vi "Intake Loop.vi"   [LabVIEW 2016]
uses:
  Robot Global Data.vi
types:
  T1 = typedef "Intake Command Cluster.ctl" = cluster{"Intake Mode":T2, "Intake Command":T3, "Intake Manual Power":dbl}
  T2 = typedef "Intake Mode.ctl" = enum16{"Manual", "Auto"}
  T3 = typedef "Intake Commands.ctl" = enum16{"Idle", "Intake", "Outtake"}
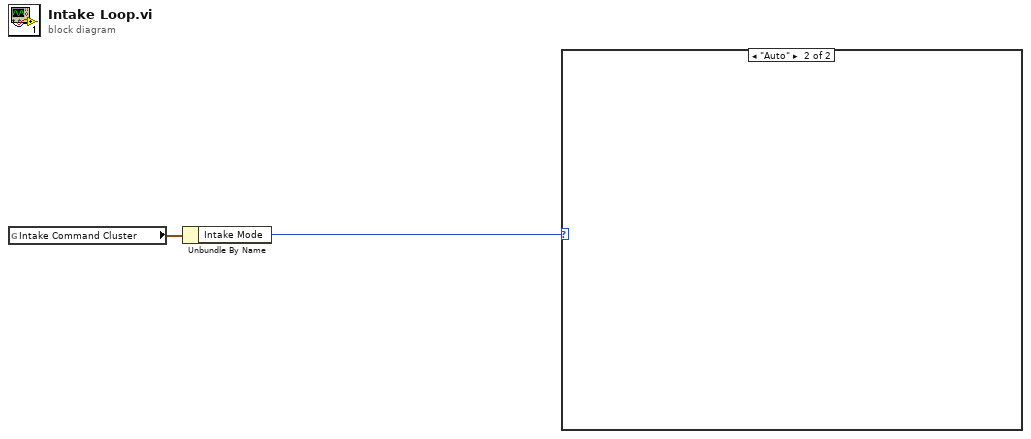
[diagram p0: block diagram]
diagram:
  n1 = global read "Robot Global Data.vi" "Intake Command Cluster"() -> (w2:T1)
  n2 = Unbundle By Name(w2) -> ("Intake Mode"=w1:T2)
  n3 = case shown="\"Auto\"" w1 {
    frame "Manual", Default {
    }
    frame "Auto" {
    }
  }
